vi "File_Get New Vi.vi"(0 "VI REF":refnum<vi>, 3 "Error":errorcluster, 4 "Path":path) -> (7 "VI REF Out":refnum<vi>, 8 "Vi Not Found Out":bool, 10 "Error Out":errorcluster)   [LabVIEW 2009]
doc: "Opens a reference to a vi if it can be found"
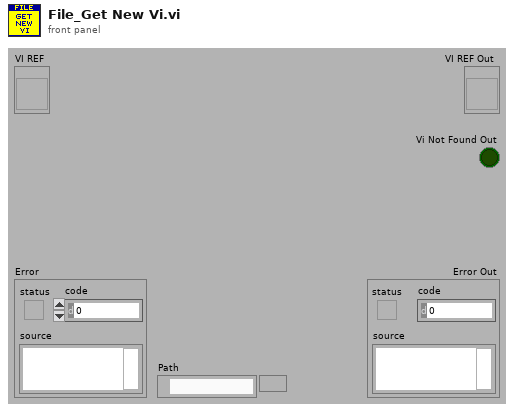
[diagram p1: front panel]
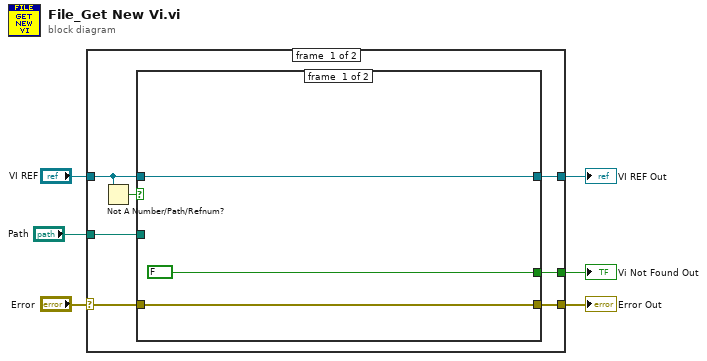
[diagram p0: block diagram]
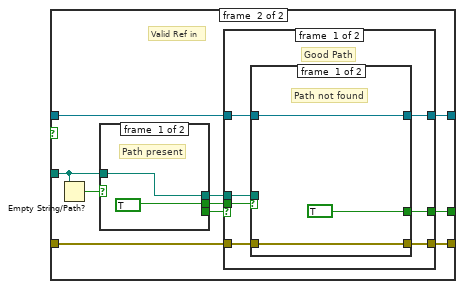
[diagram p2: hidden frame]
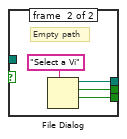
[diagram p3: hidden frame]
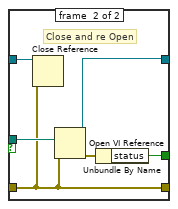
[diagram p4: hidden frame]
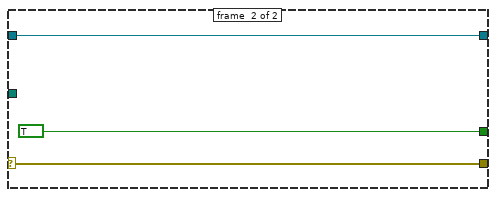
[diagram p6: hidden frame]
diagram:
  n1 = case shown="No Error" "Error" {
    selector: "Error" -> [w7 w52]
    tunnel: [w13 TRUE ("status")] -> w6
    tunnel: [w12 w54] -> w5
    tunnel: [w11 w52] -> w4
    tunnel: "VI REF" -> [w9 w54]
    tunnel: "Path" -> [w8 _]
    frame #0 {
      n2 = Not A Number/Path/Refnum?(number/path/refnum=w9) -> (NaN/Path/Refnum?=w10:bool)
      n3 = case shown="True" w10 {
        tunnel: [FALSE w26] -> w13
        tunnel: [w16 w25] -> w12
        tunnel: w9 -> [w16 w24]
        tunnel: [w15 w20] -> w11
        tunnel: w7 -> [w15 w19]
        tunnel: w8 -> [_ w17]
        frame #0 {
        }
        frame #1 {
          # "Valid Ref in"
          n4 = Empty String/Path?(string/path=w17) -> (empty?=w18:bool)
          n5 = case shown="True" w18 {
            tunnel: [_ w32] -> w23
            tunnel: [TRUE w31] -> w22
            tunnel: [w28 w30] -> w21
            tunnel: w17 -> [w28 _]
            frame #0 {
              # "Path present"
            }
            frame #1 {
              # "Empty path"
              n6 = File Dialog(7:"Select a Vi" ("prompt")) -> (1:w32:bool, 2:w31:bool, 3:w30:path)  [unwired: 6 in, 1 out]
            }
          }
          n7 = case shown="False" w23 {
            selector: w23 -> [_ w51]
            tunnel: w19 -> [w39 w50]
            tunnel: [w38 w50] -> w20
            tunnel: w21 -> [w37 _]
            tunnel: w22 -> [w36 _]
            tunnel: w24 -> [w35 w49]
            tunnel: [w34 w49] -> w25
            tunnel: [w33 w51] -> w26
            frame #0 {
              # "Good Path"
              n8 = case shown="True" w36 {
                tunnel: w39 -> [w41 w45]
                tunnel: [w41 w45] -> w38
                tunnel: w37 -> [_ w48]
                tunnel: w35 -> [w42 w47]
                tunnel: [w42 w46] -> w34
                tunnel: [TRUE w43] -> w33
                frame #0 {
                  # "Path not found"
                }
                frame #1 {
                  # "Close and re Open"
                  n9 = Close Reference(reference=w47, error in (no error)=w45) -> ()  [unwired: 1 out]
                  n10 = Open VI Reference(vi path=w48, error in (no error)=w45) -> (vi reference=w46:refnum<vi>, error out=w44:errorcluster)  [unwired: 4 in]
                  n11 = Unbundle By Name(w44) -> ("status"=w43:bool)
                }
              }
            }
            frame #1 {
              # "Bad Path"
            }
          }
        }
      }
    }
    frame #1 {
    }
  }
  "Vi Not Found Out" <- w6
  "VI REF Out" <- w5
  "Error Out" <- w4
